vi "Enable Channel Load.vi"(8 "error in (no error)":errorcluster, 11 "Device Item Ref in":T1 format="%.0x") -> (0 "error out":errorcluster, 3 "Device Item Ref out":T1 format="%.0x")   [LabVIEW 2009, in "NI-XNET Custom Device.lvlib"]
doc: "This VI is automatically called when the channel configuration is loaded. Look at the .xml file to see how to enable this VI to be called automatically."
uses:
  NI-XNET Custom Device.lvlib
  <vilib>/NI VeriStand/Custom Device API/Custom Device Item Ref.ctl
  <vilib>/NI VeriStand/Custom Device API/Set Item Property (Variant).vi
  <vilib>/NI VeriStand/Custom Device API/Get Item Property (Variant).vi
  <vilib>/NI VeriStand/Custom Device API/Custom Device API.lvlib
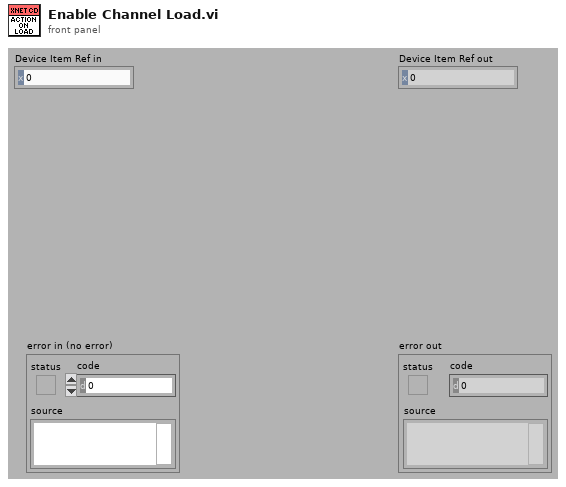
[diagram p1: front panel]
types:
  T1 = typedef "Custom Device API.lvlib/Custom Device Item Ref.ctl" = u64
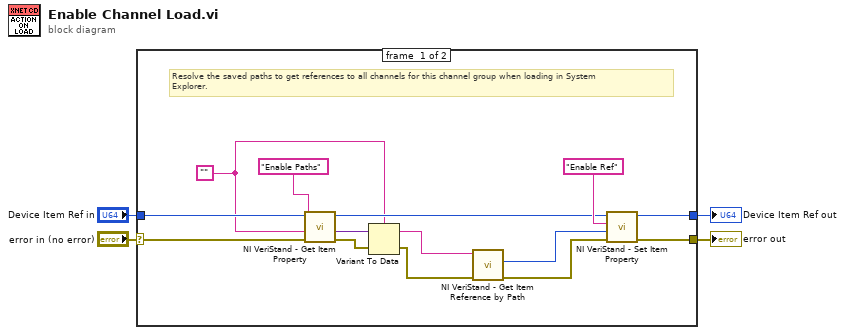
[diagram p0: block diagram]
diagram:
  n1 = case shown="No Error" "error in (no error)" {
    selector: "error in (no error)" -> [w13 w20]
    tunnel: [w7 w20] -> w3
    tunnel: "Device Item Ref in" -> [w12 w19]
    tunnel: [w6 w19] -> w1
    frame #0 {
      w5 = ""
      # "Resolve the saved paths to get references to all channels for this channel group when loading in System\nExplorer."
      n2 = call-poly <vilib>:"NI VeriStand - Get Item Property.vi"("error in (no error)"=w13, "Default Value"=w5, "Property Name"="Enable Paths", "Item Ref in"=w12) -> ("error out"=w15:errorcluster, "Value"=w16:variant, "Item Ref out"=w17:T1)  [unwired: 5 out]
      n3 = Variant To Data(error in=w15, Variant=w16, type=w5) -> (error out=w10:errorcluster, data=w11:string)
      n4 = call <vilib>:"NI VeriStand - Get Item Reference by Path.vi"("error in (no error)"=w10, "Item Path in"=w11) -> ("error out"=w8:errorcluster, "Item Ref"=w9:T1)  [unwired: 8 out]
      n5 = call-poly <vilib>:"NI VeriStand - Set Item Property.vi"("error in (no error)"=w8, "Value"=w9, "Property Name"="Enable Ref", "Item Ref in"=w17) -> ("error out"=w7:errorcluster, "Item Ref out"=w6:T1)  [unwired: 6 out]
    }
    frame #1 {
    }
  }
  "error out" <- w3
  "Device Item Ref out" <- w1
